vi "Open.vi"(4 "Permissions":T2={"Owner"={"Read"=TRUE, "Write"=TRUE, "Execute"=FALSE}, "Group"={"Read"=TRUE, "Write"=FALSE, "Execute"=FALSE}, "Others"={"Read"=TRUE, "Write"=FALSE, "Execute"=FALSE}}, 6 "Flags":T1={"Read"=TRUE, "Write"=TRUE, "Append"=FALSE, "Create"=FALSE, "Truncate"=FALSE, "Exclude"=FALSE}, 8 "Error In":errorcluster, 10 "Remote Path":string, 11 "SFTP":refnum<class "SFTP.lvclass">) -> (0 "Error Out":errorcluster, 3 "SFTP File":refnum<class "SFTP File.lvclass">)   [LabVIEW 2018, in "Toolkit.lvlib" / "SFTP File.lvclass"]
uses:
  SFTP File.lvclass
  SFTP/SFTP.lvclass
  Typedefs/Permissions.ctl
  Typedefs/Modes.ctl
  Typedefs/Flags.ctl
  SFTP/SFTP.lvclass/SFTP.ctl
  SFTP File.lvclass/SFTP File.ctl
  Toolkit.lvlib
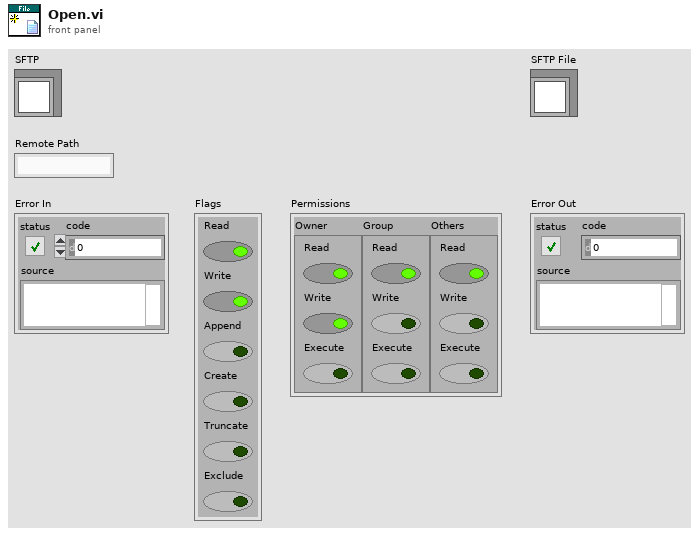
[diagram p1: front panel]
types:
  T1 = typedef "Toolkit.lvlib/SFTP File.lvclass/Flags.ctl" = cluster{"Read":bool, "Write":bool, "Append":bool, "Create":bool, "Truncate":bool, "Exclude":bool}
  T2 = typedef "Toolkit.lvlib/SFTP File.lvclass/Permissions.ctl" = cluster{"Owner":T3, "Group":T3, "Others":T3}
  T3 = typedef "Toolkit.lvlib/SFTP File.lvclass/Modes.ctl" = cluster{"Read":bool, "Write":bool, "Execute":bool}
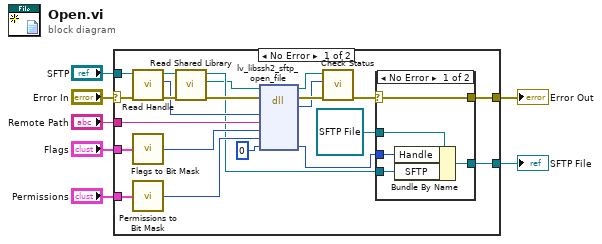
[diagram p0: block diagram]
diagram:
  n1 = case shown="No Error" "Error In" {
    selector: "Error In" -> [w23 w37]
    tunnel: [w8 w37] -> w6
    tunnel: "SFTP" -> [w24 _]
    tunnel: "Remote Path" -> [w29 _]
    tunnel: [w16 _] -> w3
    tunnel: "Permissions" -> [w15 _]
    tunnel: "Flags" -> [w13 _]
    frame No Error {
      n2 = call "Read Handle.vi"("Error In"=w23, "SFTP In"=w24) -> ("Erorr Out"=w21:errorcluster, "Handle"=w20:u64, "SFTP Out"=w22:refnum<class "SFTP.lvclass">)  [unwired: 7 in]
      n3 = call "Flags to Bit Mask.vi"("Flags"=w13) -> ("Bit Mask"=w12:u32)
      n4 = call "Permissions to Bit Mask.vi"("Permissions"=w15) -> ("Bit Mask"=w14:i32)
      n5 = call "Read Shared Library.vi"("Error In"=w21, "SFTP In"=w22) -> ("Erorr Out"=w19:errorcluster, "lv-libssh2 Shared Library"=w10:path, "SFTP Out"=w11:refnum<class "SFTP.lvclass">)  [unwired: 7 in]
      n6 = dll-call lib="D:/Users/cfield/Code/Field R&D Services/SSH/LV-LIBSSH2/LabVIEW/trunk/src/Toolkit/Support/lv-libssh2.*" fn="lv_libssh2_sftp_open_file"(path in=w10, error in=w19, "sftp"=w20, "path"=w29, "flags"=w12, "permissions"=w14, "handle"=u64 0) -> (path out=w28:path, error out=w27:errorcluster, "status"=w26:i32, "handle"=w17:u64)  [unwired: 5 in]
      n7 = call "Check Status.vi"("Error In"=w27, "Status"=w26, "lv-libssh2 Shared Library In"=w28) -> ("Error Out"=w9:errorcluster)  [unwired: 7 in, 1 out]
      n8 = case shown="No Error" w9 {
        selector: w9 -> [w30 w35]
        tunnel: refnum<class "SFTP File.lvclass"> refnum ("Toolkit.lvlib:SFTP File.lvclass") -> [w34 w36]
        tunnel: w17 -> [w33 _]
        tunnel: [w32 w36] -> w16
        tunnel: w11 -> [w31 _]
        tunnel: [w30 w35] -> w8
        frame No Error {
          n9 = Bundle By Name(cluster=w34, "Handle"=w33, "SFTP"=w31) -> (w32:refnum<class "SFTP File.lvclass">)
        }
        frame Error {
        }
      }
    }
    frame Error {
    }
  }
  "Error Out" <- w6
  "SFTP File" <- w3
